vi "Drive Distance.vi"(8 "error in":errorcluster, 9 "Auto Notifiers In":T1, 10 "Speed":dbl=0.4, 11 "Time (s)":dbl) -> (0 "error out":errorcluster, 1 "Auto Notifiers Out":T1)   [LabVIEW 2014]
uses:
  Auto Notifiers.ctl
  Main/Arms/Arm clapper state.ctl
  Main/Arms/Arm State.ctl
  Utilities/Refname.ctl
  Utilities/RefnameToString.vi
  <vilib>/Rock Robotics/WPI/RobotDrive/WPI_RobotDriveGetSetRefNum.vi
  <vilib>/Rock Robotics/WPI/RobotDrive/WPI_RobotDriveArcadeDrive_Standard(NoSaturation).vi
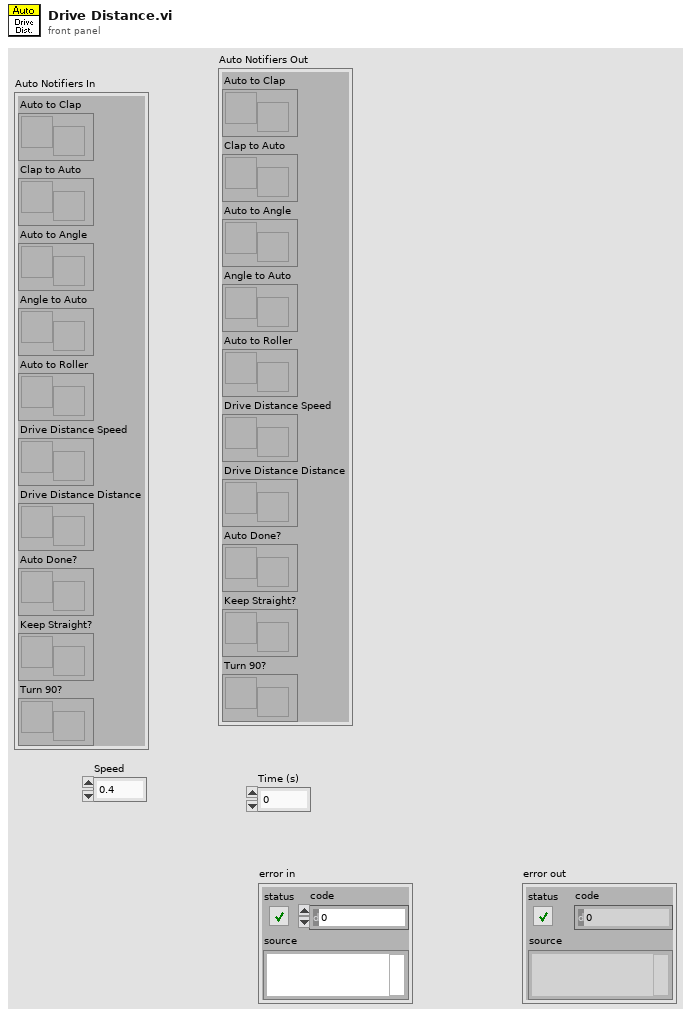
[diagram p1: front panel]
types:
  T1 = typedef "Auto Notifiers.ctl" = cluster{"Auto to Clap":refnum<notifier>, "Clap to Auto":refnum<notifier>, "Auto to Angle":refnum<notifier>, "Angle to Auto":refnum<notifier>, "Auto to Roller":refnum<notifier>, "Drive Distance Speed":refnum<notifier>, "Drive Distance Distance":refnum<notifier>, "Auto Done?":refnum<notifier>, "Keep Straight?":refnum<notifier>, "Turn 90?":refnum<notifier>}
  T2 = typedef "Refname.ctl" = enum16{"Gamepad 1", "Gamepad 2", "Drive Motors", "Strafe Motor", "Arm Clapper Motor", "Arm Angle", "Arm Belt Left", "Arm Belt Right", "Elevator 1", "Elevator 2", "Can Grabber"}
  T3 = typedef "WPI_RobotDriveDevRef.ctl" = cluster{"DevStatus":errorcluster, "Motors[]":T4[], "Square Inputs":bool, "Max Output":dbl}
  T4 = typedef "WPI_MotorControlDeviceRef.ctl" = cluster{"DeviceStatus":errorcluster, "Type":T5, "PWM":cluster{"Controller":T6, "PWM Channel":T7, "DeadBand":T8}, "CAN":cluster{"Device Number":u8, "Control Mode":T9, "Semaphore":T10, "Max Vout":dbl, "TalonSRX Control Mode":T11}, "Invert":bool, "TransformRef":T12, "InvTransformRef":T12}
  T5 = typedef "WPI_MotorControlType.ctl" = enum16{"PWM", "CAN", "CANTalonSRX"}
  T6 = typedef "FPGA_TypedefDigitalModule.ctl" = enum16{"Controller 1"}
  T7 = typedef "FPGA_DIOPWMChannel.ctl" = enum8{"PWM 0", "PWM 1", "PWM 2", "PWM 3", "PWM 4", "PWM 5", "PWM 6", "PWM 7", "PWM 8", "PWM 9", "PWM MXP 0", "PWM MXP 1", "PWM MXP 2", "PWM MXP 3", "PWM MXP 4", "PWM MXP 5", "PWM MXP 6", "PWM MXP 7", "PWM MXP 8", "PWM MXP 9", "Invalid"}
  T8 = typedef "WPI_PWMDeadband.ctl" = cluster{"Name":string, "maxPositivePwm":i32, "minPositivePwm":i32, "centerPwm":i32, "maxNegativePwm":i32, "minNegativePwm":i32, "angularRange":u16}
  T9 = typedef "WPI_CANJaguar_ControlMode.ctl" = enum8{"Percent VBus", "Current", "Speed", "Position", "Voltage"}
  T10 = typedef "Semaphore RefNum" = refnum<k1>
  T11 = typedef "WPI_CANTalonSRX_APIControlMode.ctl" = enum8{"Percent VBus", "Speed", "Position", "Slave", "Unchanged / Invalid"}
  T12 = typedef "WPI_PWMTransform_ConPane.ctl" = refnum<vi>
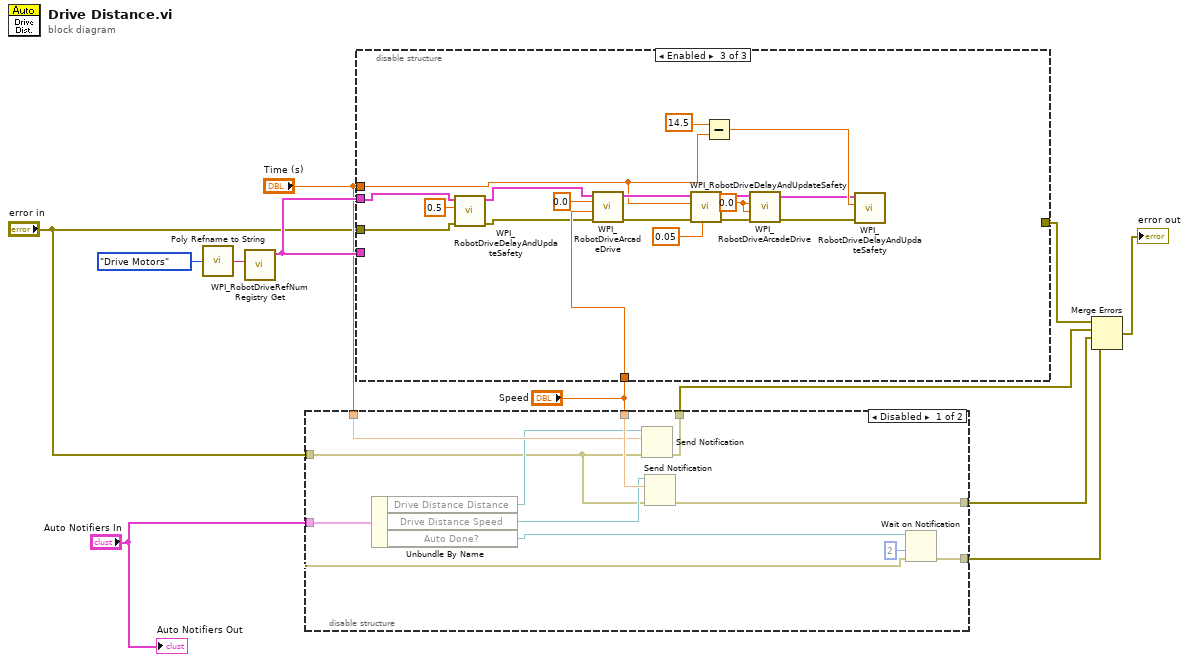
[diagram p0: block diagram]
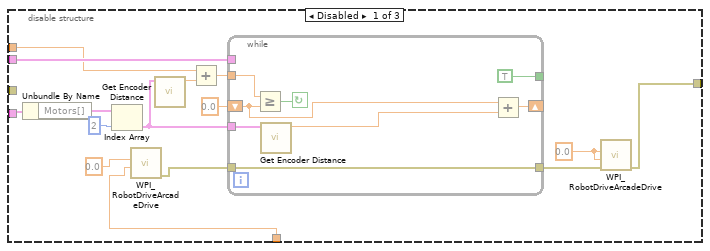
[diagram p3: hidden frame]
diagram:
  n1 = call-poly "Poly Refname to String.vi"("Enum"=Refname."Drive Motors") -> ("Refname"=w12:string)
  n2 = call <vilib>:"WPI_RobotDriveRefNum Registry Get.vi"("refnum name"=w12) -> ("RobotDriveDevRef"=w10:T3)  [unwired: 9 in, 1 out]
  n3 = disable-structure shown="Disabled" {
    disable-tunnel: "Speed" -> [w23 _]
    disable-tunnel: "Time (s)" -> [w22 _]
    disable-tunnel: "Auto Notifiers In" -> [w21 _]
    disable-tunnel: "error in" -> [w16 _]
    disable-tunnel: [w15 _] -> w3
    disable-tunnel: [w14 _] -> w2
    disable-tunnel: [w13 _] -> w1
    frame Disabled {
      n4 = Unbundle By Name(w21) -> ("Drive Distance Distance"=w20:refnum<notifier>, "Drive Distance Speed"=w19:refnum<notifier>, "Auto Done?"=w18:refnum<notifier>)
      n5 = Send Notification(notification=w22, notifier=w20, error in (no error)=w16) -> (error out=w15:errorcluster)  [unwired: 1 out]
      n6 = Send Notification(notification=w23, notifier=w19, error in (no error)=w16) -> (error out=w14:errorcluster)  [unwired: 1 out]
      n7 = Wait on Notification(notifier=w18, timeout in ms (-1)=2, error in (no error)=w16) -> (error out=w13:errorcluster)  [unwired: 1 in, 3 out]
    }
    frame Enabled {
    }
  }
  n8 = disable-structure shown="Enabled" {
    disable-tunnel: w10 -> [w25 _ _]
    disable-tunnel: w10 -> [w38 _ w53]
    disable-tunnel: "Time (s)" -> [w37 _ w49]
    disable-tunnel: "error in" -> [_ _ w56]
    disable-tunnel: [w27 _ _] -> w4
    disable-tunnel: "Speed" -> [w24 _ w59]
    frame Disabled {
      w28 = 0.0 ("X axis value")
      n9 = Unbundle By Name(w25) -> ("Motors[]"=w26:T4[])
      n10 = Index Array(array=w26, index=2) -> (element=w34:T4)
      n11 = call-poly <vilib>:"WPI_RobotDriveArcadeDrive.vi"("Y axis value"=w24, "X axis value"=0.0) -> ("error out"=w31:errorcluster)  [unwired: 7 in, 2 out]
      n12 = call "Get Encoder Distance.vi"("CAN Talon SRX Ref"=w34) -> ("Inches"=w35:dbl)  [unwired: 10 in]
      n13 = Add(x=w37, y=w35) -> (x+y=w36:dbl)
      n14 = while {
        tunnel: w36 -> [w43]
        tunnel: w38 -> [_]
        tunnel: w34 -> [w46]
        tunnel: w31 -> [w45]
        tunnel: [w45] -> w29
        shift-right: [w41] -> _
        shift-left: 0.0 ("Inches") -> [w40]
        tunnel: [TRUE] -> _
        stop <- w42 continue-if-true
        n15 = Greater Or Equal?(x=w43, y=w40) -> (x >= y?=w42:bool)
        n16 = call "Get Encoder Distance.vi"("CAN Talon SRX Ref"=w46) -> ("Inches"=w44:dbl)  [unwired: 10 in]
        n17 = Add(x=w40, y=w44) -> (x+y=w41:dbl)
      }
      n18 = call-poly <vilib>:"WPI_RobotDriveArcadeDrive.vi"("error in (no error)"=w29, "Y axis value"=w28, "X axis value"=w28) -> ("error out"=w27:errorcluster)  [unwired: 6 in, 2 out]
    }
    frame Disabled {
    }
    frame Enabled {
      w57 = 0.0 ("X axis value")
      n19 = call <vilib>:"WPI_RobotDriveDelayAndUpdateSafety.vi"("error in (no error)"=w56, "Delay (s)"=0.5, "RobotDriveDevRef"=w53) -> ("error out"=w55:errorcluster, "RobotDriveDevRef 2"=w52:T3)  [unwired: 7 in]
      n20 = call-poly <vilib>:"WPI_RobotDriveArcadeDrive.vi"("error in (no error)"=w55, "Y axis value"=w59, "X axis value"=0.0, "RobotDriveDevRef"=w52) -> ("error out"=w63:errorcluster, "RobotDriveDevRef"=w62:T3)  [unwired: 5 in, 1 out]
      n21 = call <vilib>:"WPI_RobotDriveDelayAndUpdateSafety.vi"("Feed time (s)"=0.05, "error in (no error)"=w63, "Delay (s)"=w49, "RobotDriveDevRef"=w62) -> ("error out"=w64:errorcluster, "RobotDriveDevRef 2"=w61:T3)  [unwired: 6 in]
      n22 = Subtract(x=14.5 ("Delay (s)"), y=w49) -> (x-y=w48:dbl)
      n23 = call-poly <vilib>:"WPI_RobotDriveArcadeDrive.vi"("error in (no error)"=w64, "Y axis value"=w57, "X axis value"=w57, "RobotDriveDevRef"=w61) -> ("error out"=w51:errorcluster, "RobotDriveDevRef"=w47:T3)  [unwired: 5 in, 1 out]
      n24 = call <vilib>:"WPI_RobotDriveDelayAndUpdateSafety.vi"("error in (no error)"=w51, "Delay (s)"=w48, "RobotDriveDevRef"=w47) -> ()  [unwired: 7 in, 2 out]
    }
  }
  n25 = Merge Errors(w4, w3, w2, w1) -> (→"error out":errorcluster)
  "Auto Notifiers Out" <- "Auto Notifiers In"
